vi "_tester4_.vi"() -> ()   [LabVIEW 2025]
uses:
  LabVIEWpcm.dll
panel:
  out "Cycle Time":dbl(graph)
  out "IPC":dbl(graph)
  in  "F-Seq. T= 64 step":bool=TRUE
  out "sum":u8
  in  "Stop Button":bool
  out "counrters":i32
  out "Level 2 miss Count":u64(graph)
  out "Cache Level 2 Hit Rate":dbl(graph)
  out "init":i32
  # "MUST BE RUN AS ADMINISTRATOR!!!"
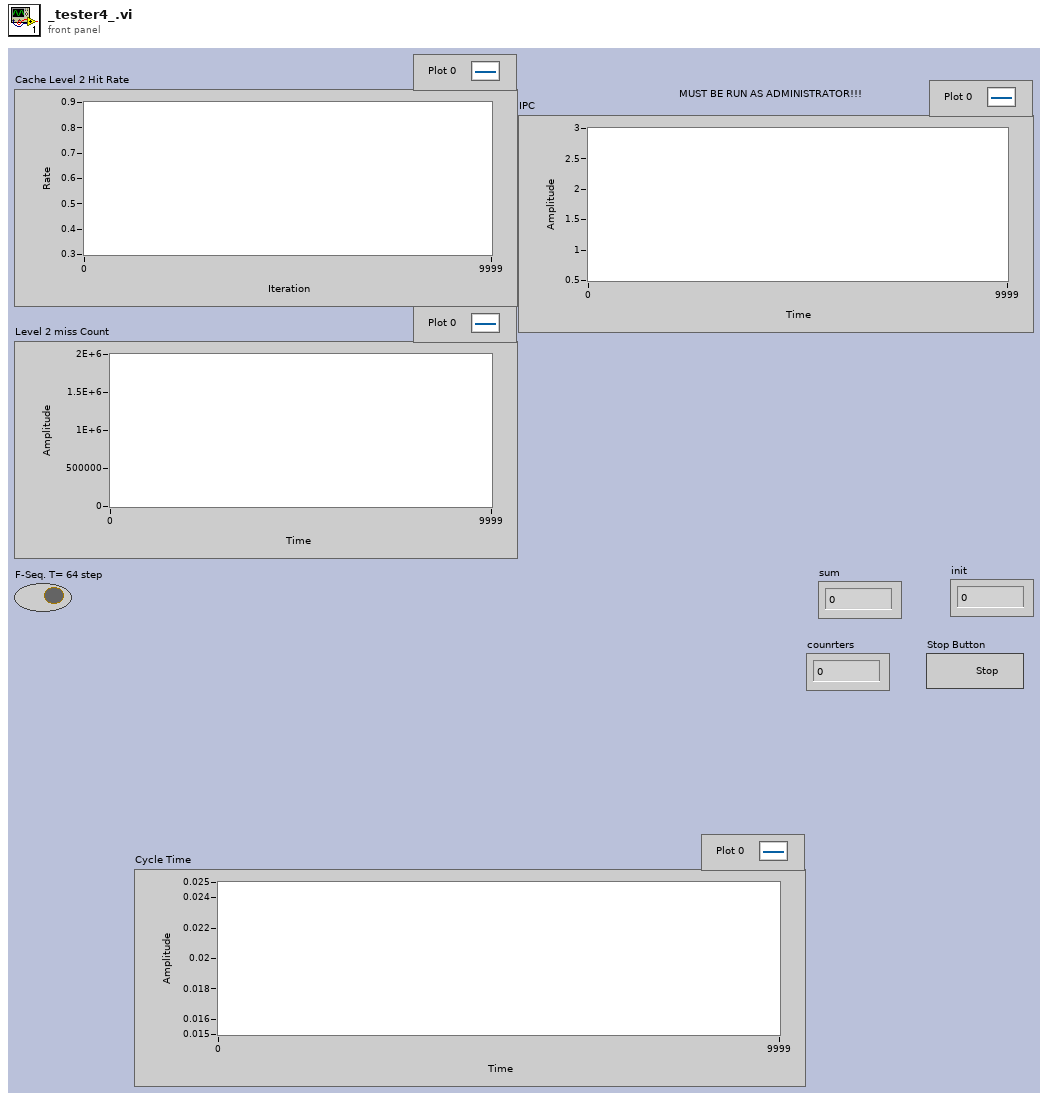
[diagram p1: front panel]
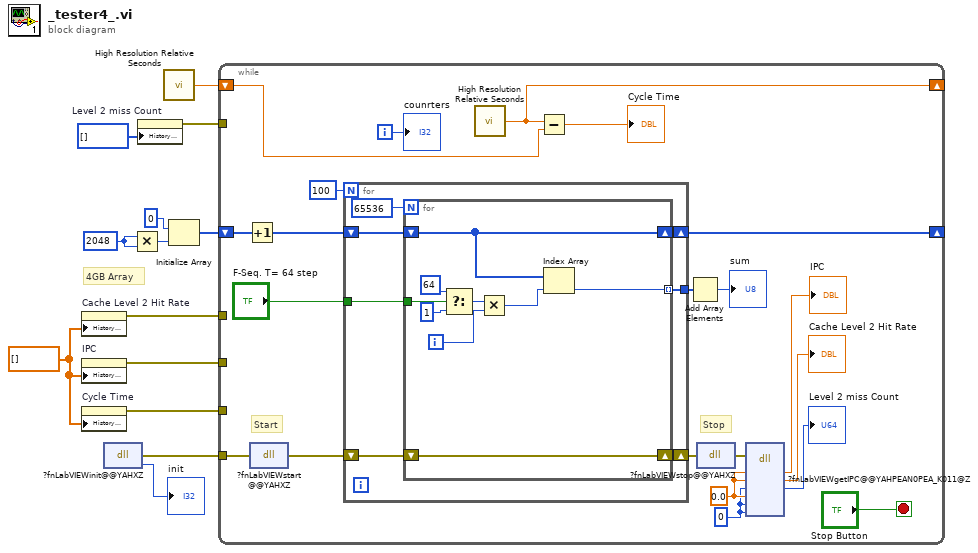
[diagram p0: block diagram]
diagram:
  w2 = dbl[] [] ("History Data")
  w5 = 2048 ("dimension size")
  # "4GB Array"
  n1 = property on="Cache Level 2 Hit Rate" class="WFChart (strict)"("History Data"=w2) -> (error out=w7:errorcluster)  [unwired: 2 in, 1 out]
  n2 = property on="IPC" class="WFChart (strict)"("History Data"=w2) -> (error out=w8:errorcluster)  [unwired: 2 in, 1 out]
  n3 = property on="Cycle Time" class="WFChart (strict)"("History Data"=w2) -> (error out=w1:errorcluster)  [unwired: 2 in, 1 out]
  n4 = dll-call lib="C:/Users/Andrey/Desktop/intel-pcm/build/x64/Release/LabVIEWpcm.dll" fn="?fnLabVIEWinit@@YAHXZ"() -> (error out=w13:errorcluster, "return type"=→"init":i32)  [unwired: 3 in, 1 out]
  n5 = Multiply(x=w5, y=w5) -> (x*y=w4:i32)
  n6 = property on="Level 2 miss Count" class="WFChart (strict)"("History Data"=u64[] []) -> (error out=w6:errorcluster)  [unwired: 2 in, 1 out]
  n7 = call <vilib>:"High Resolution Relative Seconds.vi"() -> ("relative seconds"=w3:dbl)
  n8 = Initialize Array(u8 0, w4) -> (w10:u8[])
  n9 = while {
    tunnel: w13 -> [w34]
    shift-right: [w23] -> _
    shift-left: w10 -> [w24]
    tunnel: w8 -> [_]
    tunnel: w7 -> [_]
    tunnel: w6 -> [_]
    shift-right: [w17] -> _
    shift-left: w3 -> [w19]
    tunnel: w1 -> [_]
    i -> [w28]
    stop <- "Stop Button" stop-if-true
    w31 = u64 0 ("bytes")
    w32 = 0.0 ("ipc")
    # "Stop"
    # "Start"
    n10 = Increment(x=w24) -> (x+1=w18:u8[])
    n11 = dll-call lib="C:/Users/Andrey/Desktop/intel-pcm/build/x64/Release/LabVIEWpcm.dll" fn="?fnLabVIEWstart@@YAHXZ"(error in=w34) -> (error out=w21:errorcluster)  [unwired: 3 in, 1 out]
    n12 = for {
      N: 100 -> [_]
      tunnel: [w40] -> w26
      shift-right: [w38] -> w22
      shift-left: w21 -> [w37]
      shift-right: [w39] -> w23
      shift-left: w18 -> [w36]
      tunnel: "F-Seq. T= 64 step" -> [w35]
      n13 = for {
        N: 65536 ("dimension size") -> [_]
        tunnel: [w43] -> w40 mode=indexing
        shift-right: [w50] -> w39
        shift-left: w36 -> [w50]
        shift-right: [w49] -> w38
        shift-left: w37 -> [w49]
        tunnel: w35 -> [w42]
        i -> [w48]
        n14 = Select(t=64 ("x"), s=w42, f=1 ("x")) -> (s? t:f=w45:i32)
        n15 = Multiply(x=w45, y=w48) -> (x*y=w44:i32)
        n16 = Index Array(array=w50, index=w44) -> (element=w43:u8)
      }
    }
    n17 = call <vilib>:"High Resolution Relative Seconds.vi"() -> ("relative seconds"=w17:dbl)
    n18 = Subtract(x=w17, y=w19) -> (x-y=→"Cycle Time":dbl)
    n19 = Add Array Elements(numeric array=w26) -> (sum=→"sum":u8)
    n20 = dll-call lib="C:/Users/Andrey/Desktop/intel-pcm/build/x64/Release/LabVIEWpcm.dll" fn="?fnLabVIEWstop@@YAHXZ"(error in=w22) -> (error out=w33:errorcluster)  [unwired: 3 in, 1 out]
    n21 = dll-call lib="C:/Users/Andrey/Desktop/intel-pcm/build/x64/Release/LabVIEWpcm.dll" fn="?fnLabVIEWgetIPC@@YAHPEAN0PEA_K011@Z"(error in=w33, "ipc"=w32, "lv2hit"=w32, "lv2miss"=w31, "l3hit"=w32, "l3miss"=w31, "bytes"=w31) -> ("ipc"=→"IPC":dbl, "lv2hit"=→"Cache Level 2 Hit Rate":dbl, "lv2miss"=→"Level 2 miss Count":u64)  [unwired: 6 in, 2 out]
    "counrters" <- w28
  }
